vi "Initialize Parent STEP Class Values.vi"(8 "error in (no error)":errorcluster, 11 "STEP in":T1) -> (0 "error out":errorcluster, 3 "STEP Out":T1)   [LabVIEW 2014, in "SeqLoop.lvlib"]
uses:
  TypeDefs/STEP.ctl
  TypeDefs/LogicParsedExpression.ctl
  Mimico Display/TypeDefs/Mimic Data.ctl
  Mimico Display/TypeDefs/BG Image.ctl
  Mimico Display/TypeDefs/mObject.ctl
  SeqLoop.lvlib
  Mimico Display/Mimico Display.lvlib
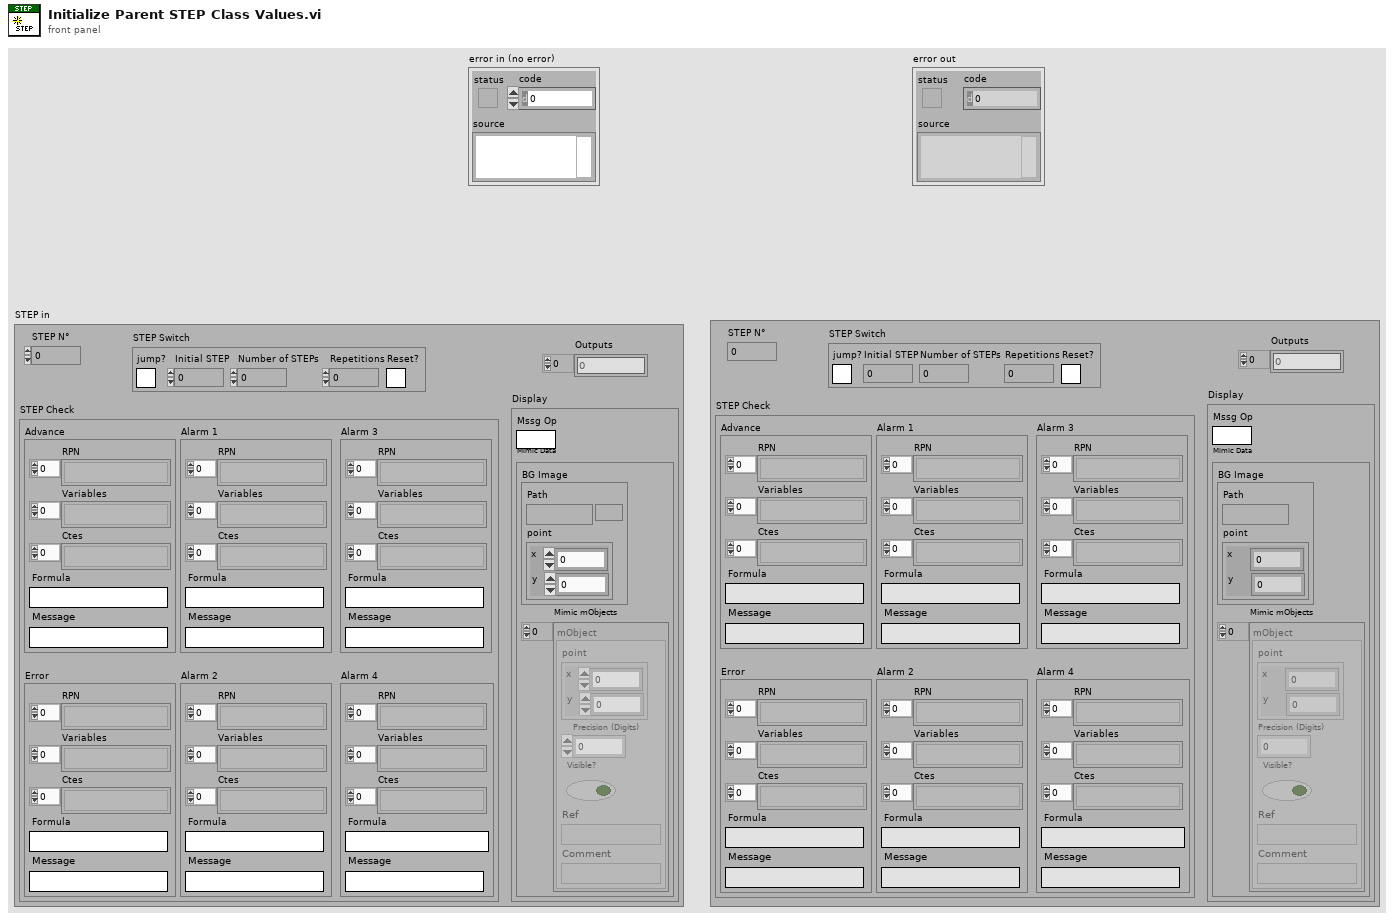
[diagram p1: front panel]
types:
  T1 = typedef "SeqLoop.lvlib/STEP.ctl" = cluster{"STEP N°":u32, "STEP Switch":cluster{"jump?":bool, "Initial STEP":u32, "Number of STEPs":u32, "Repetitions":u32, "Reset?":bool}, "Outputs":i32[], "STEP Check":cluster{"Advance":T2, "Error ":T2, "Alarm 1":T2, "Alarm 2":T2, "Alarm 3":T2, "Alarm 4":T2}, "Display":cluster{"Mssg Op":string, "Mimic Data":T3}}
  T2 = typedef "SeqLoop.lvlib/LogicParsedExpression.ctl" = cluster{"RPN ":string[], "Variables":string[], "Ctes":string[], "Formula":string, "Message":string}
  T3 = typedef "SeqLoop.lvlib/Mimico Display.lvlib/Mimic Data.ctl" = cluster{"BG Image":T4, "Mimic mObjects":T5[]}
  T4 = typedef "SeqLoop.lvlib/Mimico Display.lvlib/BG Image.ctl" = cluster{"Path":path, "point":cluster{"x":i16, "y":i16}}
  T5 = typedef "SeqLoop.lvlib/Mimico Display.lvlib/mObject.ctl" = cluster{"point":cluster{"x":i16, "y":i16}, "Precision (Digits)":i32, "Visible?":bool, "Ref":string, "Comment":string}
  T6 = cluster{"jump?":bool, "Initial STEP":u32, "Number of STEPs":u32, "Repetitions":u32, "Reset?":bool}
  T7 = cluster{"Advance":T2, "Error ":T2, "Alarm 1":T2, "Alarm 2":T2, "Alarm 3":T2, "Alarm 4":T2}
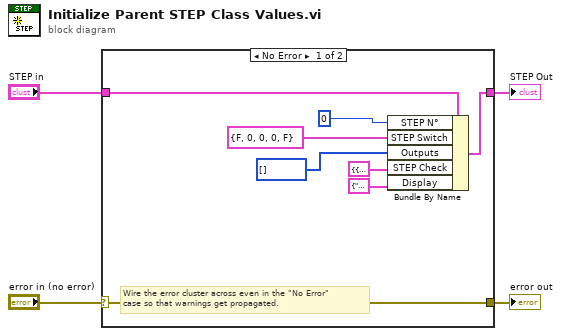
[diagram p0: block diagram]
diagram:
  n1 = case shown="No Error" "error in (no error)" {
    selector: "error in (no error)" -> [w12 w14]
    tunnel: [w12 w14] -> w3
    tunnel: [w10 w13] -> w1
    tunnel: "STEP in" -> [w11 w13]
    frame No Error {
      # "Wire the error cluster across even in the \"No Error\"\ncase so that warnings get propagated."
      n2 = Bundle By Name(cluster=w11, "STEP N°"=u32 0, "STEP Switch"=T6 {"jump?"=FALSE, "Initial STEP"=0, "Number of STEPs"=0, "Repetitions"=0, "Reset?"=FALSE}, "Outputs"=i32[] [], "STEP Check"=T7 {"Advance"={"RPN "=[], "Variables"=[], "Ctes"=[], "Formula"="", "Message"=""}, "Error "={"RPN "=[], "Variables"=[], "Ctes"=[], "Formula"="", "Message"=""}, "Alarm 1"={"RPN "=[], "Variables"=[], "Ctes"=[], "Formula"="", "Message"=""}, "Alarm 2"={"RPN "=[], "Variables"=[], "Ctes"=[], "Formula"="", "Message"=""}, "Alarm 3"={"RPN "=[], "Variables"=[], "Ctes"=[], "Formula"="", "Message"=""}, "Alarm 4"={"RPN "=[], "Variables"=[], "Ctes"=[], "Formula"="", "Message"=""}}, "Display"=cluster{"Mssg Op":string, "Mimic Data":T3} {"Mssg Op"="", "Mimic Data"={"BG Image"={"Path"=path "", "point"={"x"=0, "y"=0}}, "Mimic mObjects"=[]}}) -> (w10:T1)
    }
    frame Error {
    }
  }
  "error out" <- w3
  "STEP Out" <- w1
